vi "ModbusFrame.vi"() -> ()   [LabVIEW 2016]
uses:
  <vilib>/Instr/_visa.llb/VISA Configure Serial Port (Instr).vi
panel:
  in  "milliseconds to wait":u32
  in  "byte count":u32
  out "length":i32
  out "Bytes Read":u32
  in  "Detener Ciclo":bool
  out "Response":string
  out "Error Final":errorcluster
  in  "VISA resource name":refnum<visa-resource-name>="COM7"
  out "Request":string
  in  "Quantity":u8
  in  "Address":u8
  in  "Function Code":u8(ring) items=["Read Coils"=1, "Read Discrete Inputs"=2, "Read Holding Registers"=3, "Read Input Register"=4, "Write Single Coil"=5, "Write Single Register"=6]
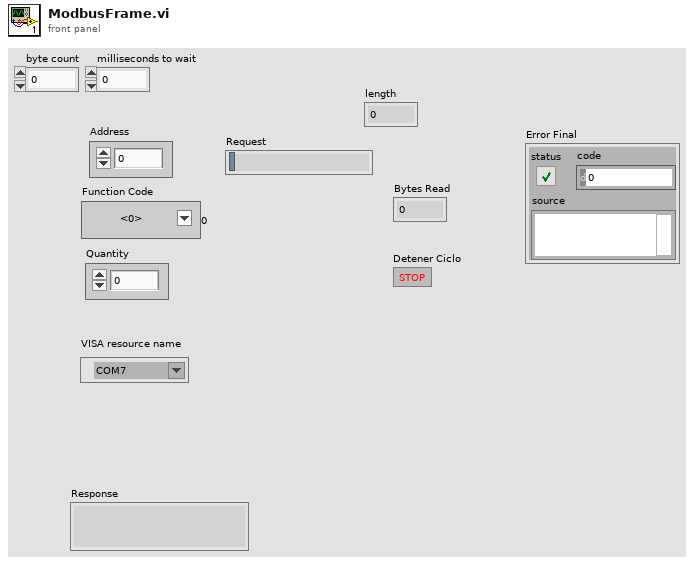
[diagram p1: front panel]
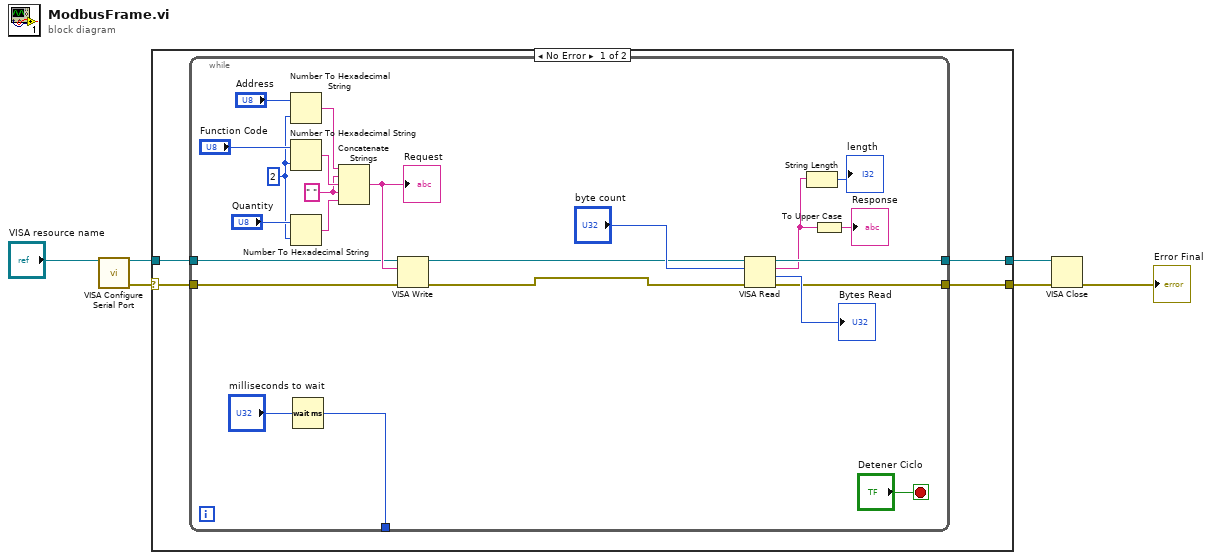
[diagram p0: block diagram]
diagram:
  n1 = call-poly "VISA Configure Serial Port"("VISA resource name"="VISA resource name") -> ("VISA resource name out"=w3:refnum<visa-resource-name>, "error out"=w4:errorcluster)  [unwired: 13 in]
  n2 = case shown="No Error" w4 {
    selector: w4 -> [w9 w35]
    tunnel: w3 -> [w8 w34]
    tunnel: [w7 w35] -> w2
    tunnel: [w10 w34] -> w1
    frame No Error {
      n3 = while {
        tunnel: [w17] -> _
        tunnel: w8 -> [w11]
        tunnel: [w24] -> w10
        tunnel: w9 -> [w25]
        tunnel: [w16] -> w7
        stop <- "Detener Ciclo" stop-if-true
        w26 = i16 2 ("width (-)")
        w28 = " "
        n4 = Number To Hexadecimal String(1:w26, 2:"Address") -> (0:w30:string)
        n5 = Number To Hexadecimal String(1:w26, 2:"Function Code") -> (0:w29:string)
        n6 = Number To Hexadecimal String(1:w26, 2:"Quantity") -> (0:w27:string)
        n7 = Wait (ms)(milliseconds to wait="milliseconds to wait") -> (millisecond timer value=w17:u32)
        n8 = Concatenate Strings(w30, w28, w29, w28, w27) -> (w23:string)
        "Request" <- w23
        n9 = VISA Write(VISA resource name=w11, write buffer=w23, error in (no error)=w25) -> (VISA resource name out=w12:refnum<visa-resource-name>, error out=w19:errorcluster)  [unwired: 1 out]
        n10 = VISA Read(VISA resource name=w12, byte count="byte count", error in (no error)=w19) -> (VISA resource name out=w24:refnum<visa-resource-name>, read buffer=w13:string, return count=→"Bytes Read":u32, error out=w16:errorcluster)
        n11 = String Length(string=w13) -> (length=→"length":i32)
        n12 = To Upper Case(1:w13) -> (0:→"Response":string)
      }
    }
    frame Error {
    }
  }
  n13 = VISA Close(VISA resource name=w1, error in (no error)=w2) -> (error out=→"Error Final":errorcluster)
